vi "Returning Values By Reference 2D Array Of Integers.vi"(9 "newArray":i32, 10 "cols":i32, 11 "rows":i32) -> (1 "newArray out":i32)   [LabVIEW 2018, in "ParsingDataSampleDLL.lvlib"]
doc: "__declspec(dllexport) void ReturningValuesByReference_2DArrayOfIntegers (int rows, int cols, int ***newArray);"
uses:
  ParsingDataSampleDLL.lvlib
  ni_reference_vs/Debug/ParsingDataSampleDLL.dll
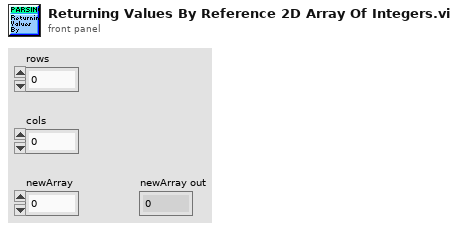
[diagram p1: front panel]
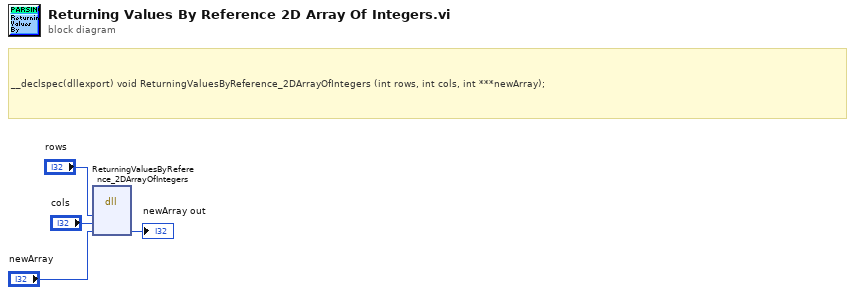
[diagram p0: block diagram]
diagram:
  # "__declspec(dllexport) void ReturningValuesByReference_2DArrayOfIntegers (int rows, int cols, int ***newArray);"
  n1 = dll-call lib="C:/Users/celit/Documents/GitHub/Labview_Python_DLL_Call/ni_reference_vs/Debug/ParsingDataSampleDLL.*" fn="ReturningValuesByReference_2DArrayOfIntegers"("rows"="rows", "cols"="cols", "newArray"="newArray") -> ("newArray"=→"newArray out":i32)  [unwired: 6 in, 2 out]
